vi "FunctionGenerator_Execute.vi"(7 "X Y Pairs":T1[](array[typedef]) {"Y" format="%_7f"; "X" format="%_7f"}, 11 "Input Value":dbl) -> (3 "Output Value":dbl)   [LabVIEW 2019, in "Trajectory_Library.lvlib"]
doc: "Convience, single call, LabVIEW function. Creates and calculates the function generator.\n\n\nInputs:\n\nOutputs:"
uses:
  Trajectory_Library.lvlib
  X_Y_PAIR.ctl
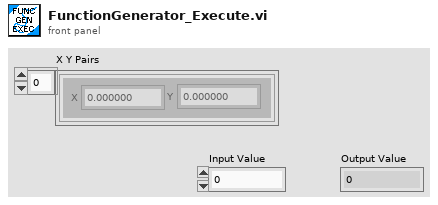
[diagram p1: front panel]
types:
  T1 = typedef "Trajectory_Library.lvlib/X_Y_PAIR.ctl" = cluster{"X":dbl, "Y":dbl}
  T2 = typedef "Trajectory_Library.lvlib/FUNCTION_GENERATOR.ctl" = cluster{"MinX":dbl, "MaxX":dbl, "ItemCount":i32, "Table Ys":dbl[], "Table Xs":dbl[]}
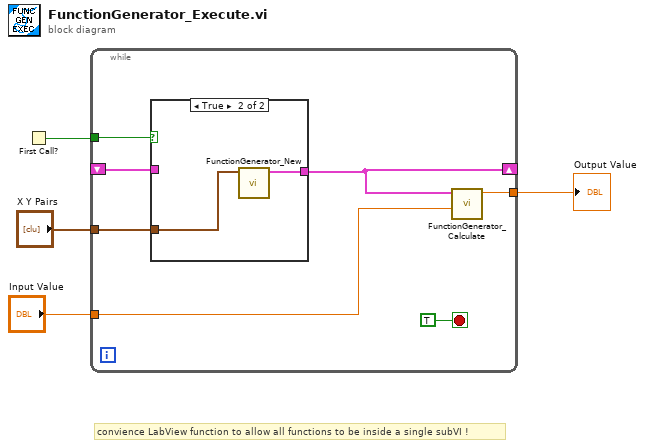
[diagram p0: block diagram]
diagram:
  # "convience LabView function to allow all functions to be inside a single subVI !"
  n1 = First Call?() -> (First Call?: T/F=w4:bool)
  n2 = while {
    shift-right: [w7] -> _
    shift-left: _ -> [w11]
    tunnel: w4 -> [w9]
    tunnel: "X Y Pairs" -> [w8]
    tunnel: "Input Value" -> [w6]
    tunnel: [w5] -> w1
    stop <- TRUE stop-if-true
    n3 = case shown="True" w9 {
      tunnel: w11 -> [w12 _]
      tunnel: [w12 w14] -> w7
      tunnel: w8 -> [_ w13]
      frame False {
      }
      frame True {
        n4 = call "FunctionGenerator_New.vi"("X Y Pairs"=w13) -> ("FUNCTION_GENERATOR"=w14:T2)  [unwired: 10 in]
      }
    }
    n5 = call "FunctionGenerator_Calculate.vi"("Input Value"=w6, "FUNCTION_GENERATOR"=w7) -> ("Output Value"=w5:dbl)  [unwired: 9 in]
  }
  "Output Value" <- w1
